vi "testAddStatesToQueueWhitespaceHandling3.vi"(8 "error in (no error)":errorcluster, 11 "testStateMachineUtilities in":refnum<class "testStateMachineUtilities.lvclass">=refnum) -> (0 "error out":errorcluster, 3 "testStateMachineUtilities out":refnum<class "testStateMachineUtilities.lvclass">)   [LabVIEW 2016, in "testStateMachineUtilities.lvclass"]
uses:
  testStateMachineUtilities.lvclass
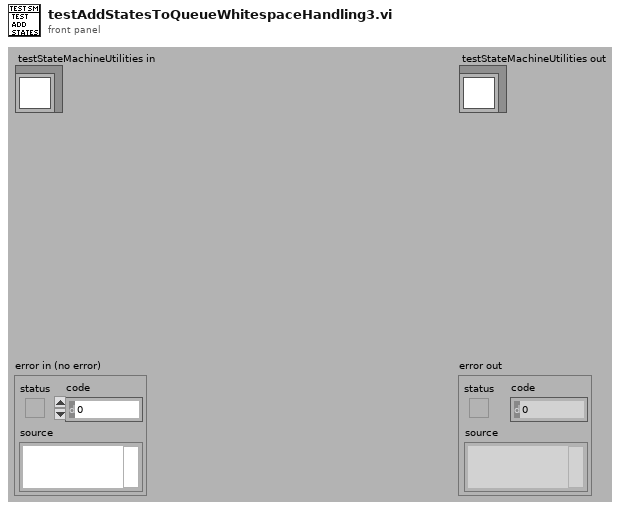
[diagram p1: front panel]
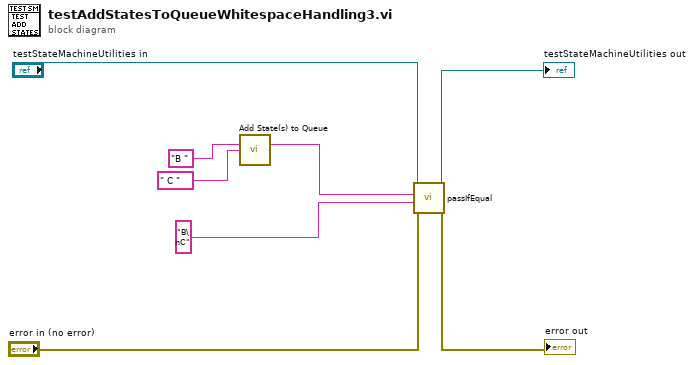
[diagram p0: block diagram]
diagram:
  n1 = call "Add State(s) to Queue.vi"("State(s) in (\"\")"="B " ("State(s) in"), "State(s) at Back (\"\")"=" C " ("State(s) in")) -> ("States Out"=w6:string)  [unwired: 13 in]
  n2 = call-dynamic "passIfEqual.vi"("error in (no error)"="error in (no error)", "y"="B\nC" ("State(s) at Back"), "x"=w6, "TestCase in"="testStateMachineUtilities in") -> ("error out"=→"error out":errorcluster, "TestCase out"=→"testStateMachineUtilities out":refnum<class "testStateMachineUtilities.lvclass">)  [unwired: 6 in]
